vi "BuildDescription.vi"(2 "MyState":T1, 3 "ROS in":T2={"topic port"=1236, "Node"="/labview", "topic"="/robot/head/command_head_nod", "type"="std_msgs/Bool", "node port"=7000, "error "={"status"=FALSE, "code"=0, "source"=""}, "Direction"=enum."Publisher", "Update (ms)"=1, "FIFO size"=1}) -> (1 "Setup":string)   [LabVIEW 2016]
doc: "Builds a description from ROS definitions"
uses:
  SubVIs/_ROSControl.ctl
  SubVIs/_ROSDirection.ctl
  MyState.ctl
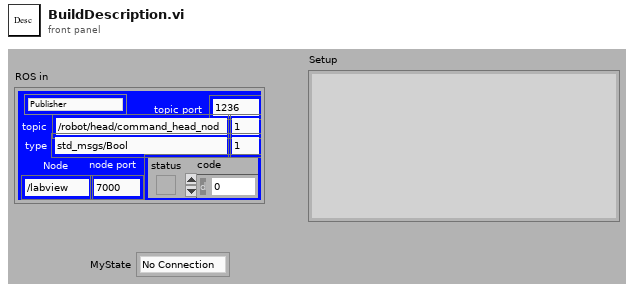
[diagram p1: front panel]
types:
  T1 = typedef "MyState.ctl" = enum16{"No Connection", "Registered", "Connected", "Close"}
  T2 = typedef "_ROSControl.ctl" = cluster{"topic port":u16, "Node":string, "topic":string, "type":string, "node port":u16, "error ":errorcluster, "Direction":T3, "Update (ms)":u16, "FIFO size":u16}
  T3 = typedef "_ROSDirection.ctl" = enum16{"Node", "Publisher", "Subscriber", "ServiceClient", "ServiceProvider"}
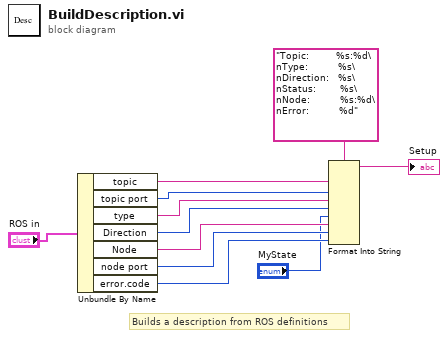
[diagram p0: block diagram]
diagram:
  # "Builds a description from ROS definitions"
  n1 = Unbundle By Name("ROS in") -> ("topic"=w10:string, "topic port"=w9:u16, "type"=w8:string, "Direction"=w7:T3, "Node"=w3:string, "node port"=w6:u16, "error.code"=w5:i32)
  n2 = Format Into String(format string="Topic:         %s:%d\nType:          %s\nDirection:   %s\nStatus:        %s\nNode:          %s:%d\nError:          %d", w10, w9, w8, w7, "MyState", w3, w6, w5) -> (resulting string=→"Setup":string)  [unwired: 2 in, 1 out]
